vi "isFull.vi"(8 "error in (no error)":errorcluster, 11 "Bucket in":refnum<class "Bucket.lvclass">) -> (0 "error out":errorcluster, 2 "Full?":bool, 3 "Bucket out":refnum<class "Bucket.lvclass">)   [LabVIEW 2017, in "Bucket.lvclass"]
uses:
  <userlib>/836-Library/Data_Structures/HashMap/Support/Bucket/Bucket.lvclass
  <userlib>/836-Library/Data_Structures/HashMap/Support/Bucket/Bucket.lvclass/Bucket.ctl
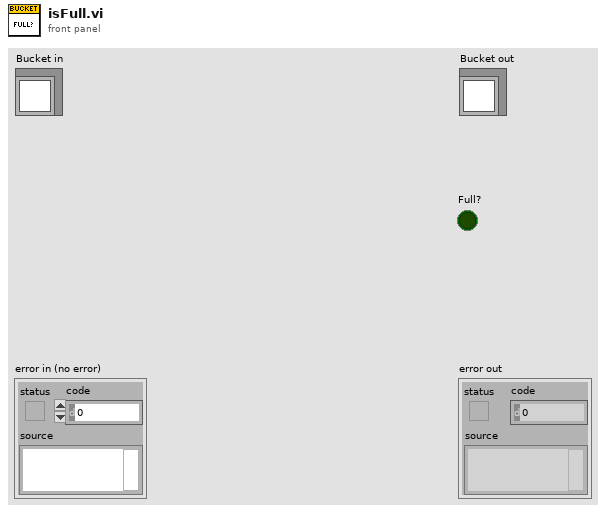
[diagram p1: front panel]
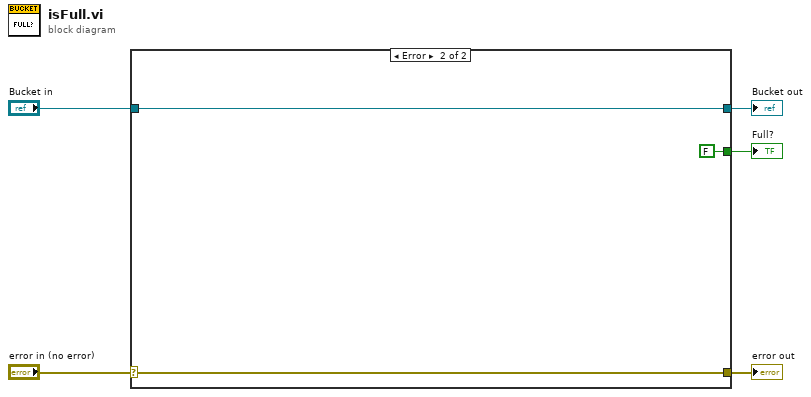
[diagram p0: block diagram]
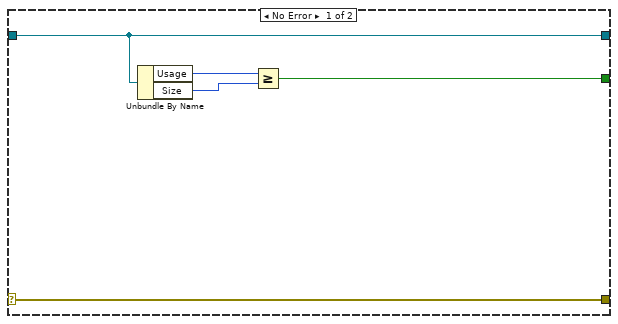
[diagram p2: hidden frame]
diagram:
  n1 = case shown="Error" "error in (no error)" {
    selector: "error in (no error)" -> [w10 w13]
    tunnel: [w10 w13] -> w4
    tunnel: [w9 w12] -> w2
    tunnel: "Bucket in" -> [w9 w12]
    tunnel: [w6 FALSE] -> w1
    frame No Error {
      n2 = Unbundle By Name(w9) -> ("Usage"=w8:u32, "Size"=w7:u32)
      n3 = Greater Or Equal?(x=w8, y=w7) -> (x >= y?=w6:bool)
    }
    frame Error {
    }
  }
  "error out" <- w4
  "Bucket out" <- w2
  "Full?" <- w1
